vi "AutoApproach.vi"() -> (2 "Surface Location (m)":dbl)   [LabVIEW 2021]
doc: "Programming Interface Example: Automatic approach implemented using Nanonis Programming Interface functions. This can be used if you want to execute special functions after each motor step or if you want to control your motor directly from LabVIEW.\n\n- Nanonis Programming Interface -"
uses:
  Program Files/National Instruments/LabVIEW 2022/user.lib/Nanonis Prog Interface V5/Nanonis Prog Interface.lvlib
panel:
  in  "stop":bool
  out "Surface reached":bool
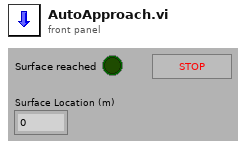
[diagram p1: front panel]
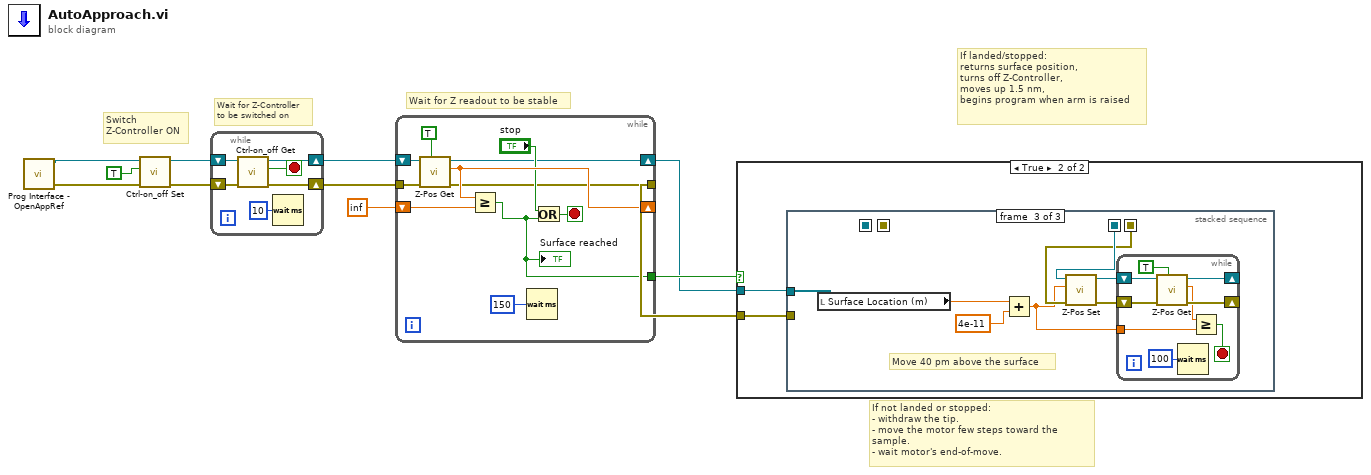
[diagram p0: block diagram]
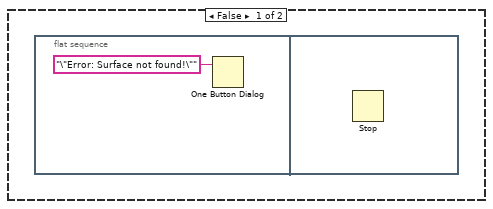
[diagram p2: hidden frame]
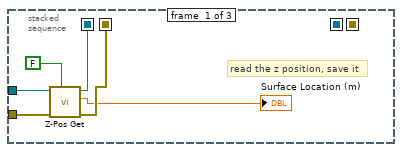
[diagram p3: hidden frame]
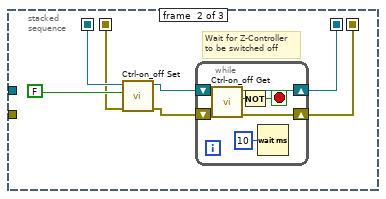
[diagram p4: hidden frame]
diagram:
  # "Wait for Z readout to be stable"
  # "If landed/stopped:  \nreturns surface position, \nturns off Z-Controller, \nmoves up 1.5 nm,\nbegins program when arm is raised"
  # "Wait for Z-Controller\nto be switched on"
  # "Switch Z-Controller ON"
  # "If not landed or stopped:\n- withdraw the tip.\n- move the motor few steps toward the sample.\n- wait motor's end-of-move."
  n1 = call <userlib>:"Prog Interface - OpenAppRef.vi"() -> ("Error out"=w10:errorcluster, "Application reference"=w11:refnum<vi>)  [unwired: 6 in]
  n2 = call <userlib>:"Ctrl-on_off Set.vi"("error in (no error)"=w10, "Z Controller ON/OFF"=TRUE ("Ctrl on/off"), "Application ref in"=w11) -> ("error out"=w6:errorcluster, "Application ref out"=w4:refnum<vi>)  [unwired: 7 in]
  n3 = while {
    shift-right: [w17] -> w5
    shift-left: w6 -> [w16]
    shift-right: [w12] -> w3
    shift-left: w4 -> [w13]
    stop <- w15 stop-if-true
    n4 = call <userlib>:"Ctrl-on_off Get.vi"("error in (no error)"=w16, "Application ref in"=w13) -> ("error out"=w17:errorcluster, "Z-Controller on/off status"=w15:bool, "Application ref out"=w12:refnum<vi>)  [unwired: 7 in]
    n5 = Wait (ms)(milliseconds to wait=u32 10) -> ()  [unwired: 1 out]
  }
  n6 = while {
    shift-right: [w26] -> _
    shift-left: sgl inf ("Z-pos (m)") -> [w28]
    tunnel: [w20] -> w9
    tunnel: w5 -> [w24]
    shift-right: [w22] -> w2
    shift-left: w3 -> [w23]
    tunnel: [w19] -> w1
    stop <- w21 stop-if-true
    n7 = call <userlib>:"Z-Pos Get.vi"("Wait for newest data (F=False)"=TRUE, "error in (no error)"=w24, "Application ref in"=w23) -> ("error out"=w19:errorcluster, "Z position (m)"=w26:sgl, "Application ref out"=w22:refnum<vi>)  [unwired: 6 in]
    n8 = Greater Or Equal?(x=w26, y=w28) -> (x >= y?=w20:bool)
    "Surface reached" <- w20
    n9 = Wait (ms)(milliseconds to wait=u32 150) -> ()  [unwired: 1 out]
    n10 = Or(x="stop", y=w20) -> (x .or. y?=w21:bool)
  }
  n11 = case shown="True" w9 {
    tunnel: w2 -> [_ w31]
    tunnel: w1 -> [_ w30]
    frame False {
      n12 = flat-sequence {
        frame #0 {
          n13 = One Button Dialog(message="\"Error: Surface not found!\"") -> ()  [unwired: 1 in, 1 out]
        }
        frame #1 {
          n14 = Stop() -> ()  [unwired: 1 in]
        }
      }
    }
    frame True {
      n15 = stacked-sequence {
        seq-local: [w37 _ _] -> [_ w43 _]
        seq-local: [w35 _ _] -> [_ w42 _]
        seq-local: [_ w39 _] -> [_ _ w57]
        seq-local: [_ w38 _] -> [_ _ w56]
        tunnel: w31 -> [w36 _ _]
        tunnel: w30 -> [w34 _ _]
        frame #0 {
          # "read the z position, save it"
          n16 = call <userlib>:"Z-Pos Get.vi"("Wait for newest data (F=False)"=FALSE, "error in (no error)"=w34, "Application ref in"=w36) -> ("error out"=w35:errorcluster, "Z position (m)"=→"Surface Location (m)":sgl, "Application ref out"=w37:refnum<vi>)  [unwired: 6 in]
        }
        frame #1 {
          # "Wait for Z-Controller\nto be switched off"
          n17 = call <userlib>:"Ctrl-on_off Set.vi"("error in (no error)"=w42, "Z Controller ON/OFF"=FALSE, "Application ref in"=w43) -> ("error out"=w40:errorcluster, "Application ref out"=w41:refnum<vi>)  [unwired: 7 in]
          n18 = while {
            shift-right: [w51] -> w38
            shift-left: w40 -> [w50]
            shift-right: [w46] -> w39
            shift-left: w41 -> [w47]
            stop <- w45 stop-if-true
            n19 = call <userlib>:"Ctrl-on_off Get.vi"("error in (no error)"=w50, "Application ref in"=w47) -> ("error out"=w51:errorcluster, "Z-Controller on/off status"=w49:bool, "Application ref out"=w46:refnum<vi>)  [unwired: 7 in]
            n20 = Not(x=w49) -> (.not. x?=w45:bool)
            n21 = Wait (ms)(milliseconds to wait=u32 10) -> ()  [unwired: 1 out]
          }
        }
        frame #2 {
          # "Move 40 pm above the surface"
          n22 = local read "Surface Location (m)"() -> (w52:dbl)
          n23 = Add(x=w52, y=4e-11) -> (x+y=w53:dbl)
          n24 = call <userlib>:"Z-Pos Set.vi"("error in (no error)"=w56, "Z position (m)"=w53, "Application ref in"=w57) -> ("error out"=w54:errorcluster, "Application ref out"=w55:refnum<vi>)  [unwired: 7 in]
          n25 = while {
            shift-right: [w64] -> _
            shift-left: w54 -> [w66]
            shift-right: [w65] -> _
            shift-left: w55 -> [w67]
            tunnel: w53 -> [w61]
            stop <- w63 stop-if-true
            n26 = call <userlib>:"Z-Pos Get.vi"("Wait for newest data (F=False)"=TRUE, "error in (no error)"=w66, "Application ref in"=w67) -> ("error out"=w64:errorcluster, "Z position (m)"=w62:sgl, "Application ref out"=w65:refnum<vi>)  [unwired: 6 in]
            n27 = Wait (ms)(milliseconds to wait=u32 100) -> ()  [unwired: 1 out]
            n28 = Greater Or Equal?(x=w62, y=w61) -> (x >= y?=w63:bool)
          }
        }
      }
    }
  }
